vi "autofile.vi"() -> ()   [LabVIEW 2018]
panel:
  out "error out":errorcluster
  in  "error in":errorcluster
  in  "File Directory":path
  out "refnum":refnum<file>
  out "Output Directory":path
  in  "Filename":string
  # "Open Directory"
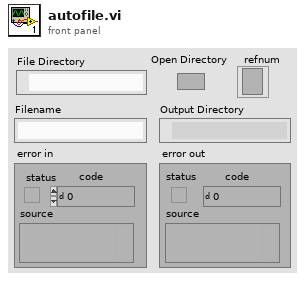
[diagram p1: front panel]
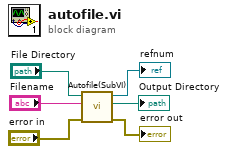
[diagram p0: block diagram]
diagram:
  n1 = call "Autofile(SubVI).vi"("error in (no error)"="error in", "Filename"="Filename", "File Directory"="File Directory") -> ("error out"=→"error out":errorcluster, "Output Directory"=→"Output Directory":path, "Byte Stream File out"=→"refnum":refnum<file>)  [unwired: 6 in]
